vi "Set Shake.vi"(8 "error in (no error)":errorcluster, 9 "Shake Amplitude (g)":dbl, 10 "Shake Frequency (Hz)":dbl, 11 "Shaker Controller in":refnum<class "Shaker Controller.lvclass">) -> (0 "error out":errorcluster, 3 "Shaker Controller out":refnum<class "Shaker Controller.lvclass">)   [LabVIEW 2020, in "Shaker Controller.lvlib" / "Shaker Controller.lvclass"]
uses:
  Shaker Controller.lvclass
  Shaker Controller.lvclass/Shaker Controller.ctl
  _Abstract Classes/Abstract Shaker/Abstract Shaker.lvclass
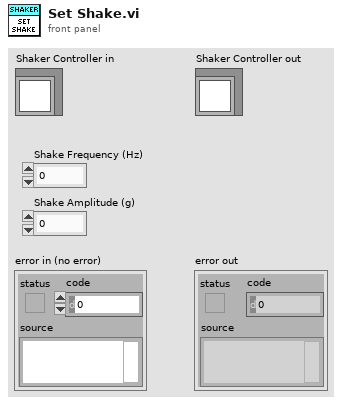
[diagram p1: front panel]
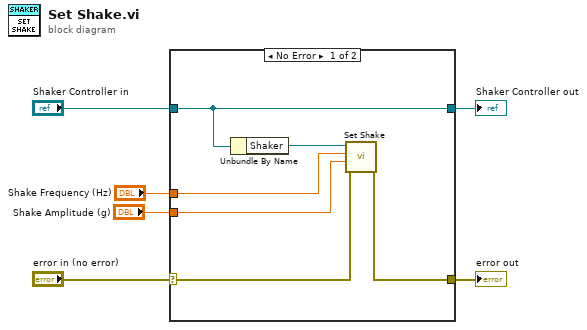
[diagram p0: block diagram]
diagram:
  n1 = case shown="No Error" "error in (no error)" {
    selector: "error in (no error)" -> [w10 w14]
    tunnel: [w9 w14] -> w5
    tunnel: [w12 w13] -> w3
    tunnel: "Shaker Controller in" -> [w12 w13]
    tunnel: "Shake Frequency (Hz)" -> [w8 _]
    tunnel: "Shake Amplitude (g)" -> [w7 _]
    frame No Error {
      n2 = Unbundle By Name(w12) -> ("Shaker"=w11:refnum<class "Abstract Shaker.lvclass">)
      n3 = call-dynamic "Set Shake.vi"("error in (no error)"=w10, "Shake Amplitude (g)"=w7, "Shake Frequency (Hz)"=w8, "Abstract Shaker in"=w11) -> ("error out"=w9:errorcluster)  [unwired: 6 in, 1 out]
    }
    frame Error {
    }
  }
  "error out" <- w5
  "Shaker Controller out" <- w3
